vi "Stop Core.vi"(10 "final error code":i32, 11 "Capillary in":refnum<class "Capillary.lvclass">) -> (3 "Capillary out":refnum<class "Capillary.lvclass">)   [LabVIEW 2015, in "AMS UI.lvlib" / "Capillary.lvclass"]
doc: "(<B>Filename</B>: Actor Framework.lvlib:Actor.lvclass:Stop Core.vi)\n\nDefines what the actor does before it stops. Use the <B>final error code</B> input to determine whether the actor shut down in response to an error.\n\nBy default, this method does nothing. A descendant class may override it to define behavior, such as shutting down any processes the actor initiated in its override of the Actor Core method."
uses:
  Capillary.lvclass
  Capillary.lvclass/Capillary.ctl
  AMS Gas Actor/AMS Gas Actor.lvclass
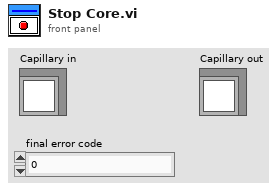
[diagram p1: front panel]
types:
  T1 = typedef "Sample Container.ctl" = cluster{"Sample In":refnum<k21>, "Sample Name":refnum<k21>, "Ti Cathode":refnum<k21>, "SampleQ":refnum<queue>}
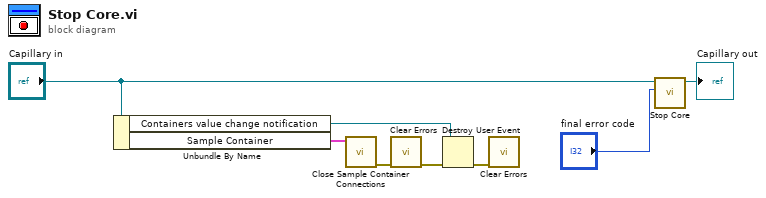
[diagram p0: block diagram]
diagram:
  n1 = Unbundle By Name("Capillary in") -> ("Containers value change notification"=w3:refnum<user-event>, "Sample Container"=w6:T1)
  n2 = call "Close Sample Container Connections.vi"("Container in"=w6) -> ("error out"=w5:errorcluster)  [unwired: 9 in, 1 out]
  n3 = call <vilib>:"Clear Errors.vi"("error in (no error)"=w5) -> ("error out"=w4:errorcluster)  [unwired: 5 in, 1 out]
  n4 = Destroy User Event(user event=w3, error in=w4) -> (error out=w2:errorcluster)
  n5 = call <vilib>:"Clear Errors.vi"("error in (no error)"=w2) -> ()  [unwired: 5 in, 2 out]
  n6 = call-parent "Stop Core.vi"("final error code"="final error code", "AMS Gas Actor in"="Capillary in") -> ("AMS Gas Actor out"=→"Capillary out":refnum<class "Capillary.lvclass">)  [unwired: 9 in]
